vi "launched.vi"   [LabVIEW 2020]
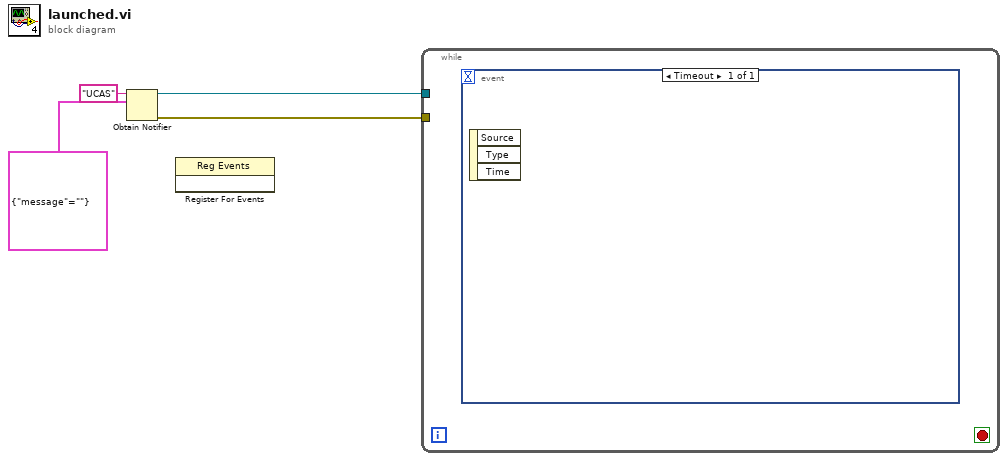
[diagram p0: block diagram]
diagram:
  n1 = Obtain Notifier(name (unnamed)="UCAS", notification data type=cluster{"message":string} {"message"=""}) -> (notifier out=w2:refnum<notifier>, error out=w1:errorcluster)  [unwired: 2 in, 1 out]
  n2 = register-events() -> ()  [unwired: 3 in, 2 out]
  n3 = while {
    tunnel: w2 -> [_]
    tunnel: w1 -> [_]
    stop <- _ stop-if-true
    n4 = event shown="[0] Timeout" {
      selector: _ -> [_]
      dyn-events: _ -> [_]
      timeout: _ -> [_]
      event Timeout {
        n5 = event-data() -> ()  [unwired: 1 in, 3 out]
      }
    }
  }
